vi "Read Sum.vi"(8 "error in (no error)":errorcluster, 11 "SimpleAdder in":refnum<class "SimpleAdder.lvclass">) -> (0 "error out":errorcluster, 2 "Sum":dbl, 3 "SimpleAdder out":refnum<class "SimpleAdder.lvclass">)   [LabVIEW 2012, in "SimpleAdder.lvclass"]
uses:
  SimpleAdder.lvclass
  SimpleAdder.lvclass/SimpleAdder.ctl
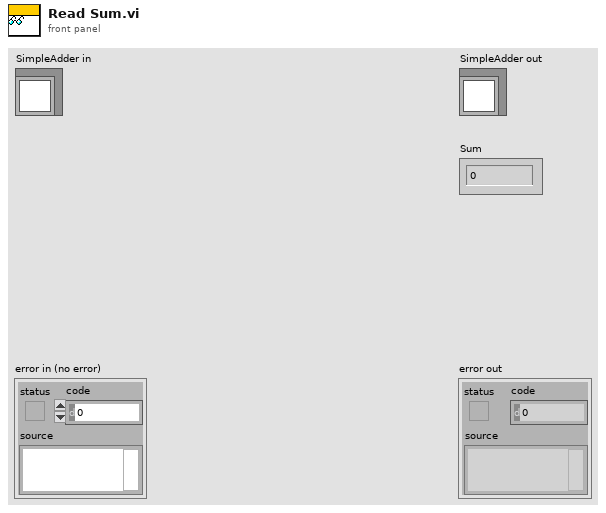
[diagram p1: front panel]
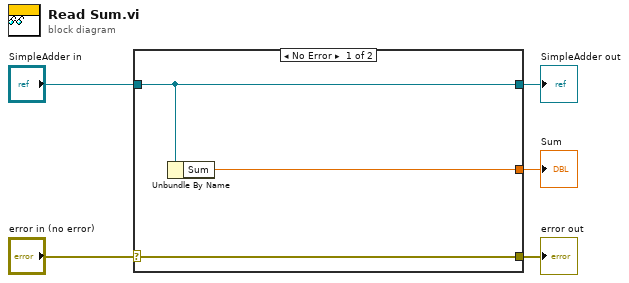
[diagram p0: block diagram]
diagram:
  n1 = case shown="No Error" "error in (no error)" {
    selector: "error in (no error)" -> [w8 w9]
    tunnel: [w8 w9] -> w4
    tunnel: [w7 w10] -> w2
    tunnel: "SimpleAdder in" -> [w7 w10]
    tunnel: [w6 _] -> w1
    frame No Error {
      n2 = Unbundle By Name(w7) -> ("Sum"=w6:dbl)
    }
    frame Error {
    }
  }
  "error out" <- w4
  "SimpleAdder out" <- w2
  "Sum" <- w1
